vi "文字转语音.vi"(8 "错误输入（无错误）":errorcluster, 11 "textToSpeak":string="急停") -> (0 "错误输出":errorcluster)   [LabVIEW 2020]
uses:
  System.Speech
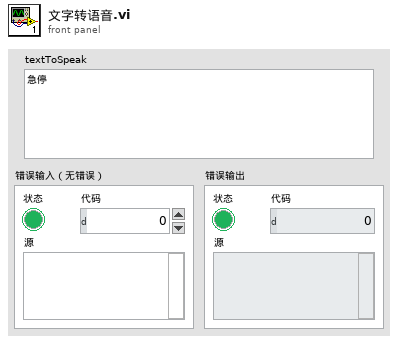
[diagram p1: front panel]
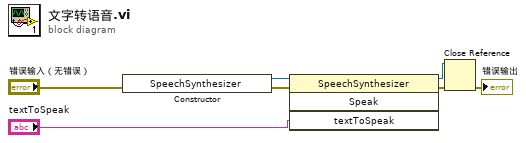
[diagram p0: block diagram]
diagram:
  n1 = constructor class="SpeechSynthesizer"(error in="错误输入（无错误）") -> (reference out=w7:refnum<k24>, error out=w3:errorcluster)  [unwired: 2 in, 1 out]
  n2 = invoke class="SpeechSynthesizer" method="Speak"(reference=w7, error in=w3, "textToSpeak"="textToSpeak") -> (reference out=w4:refnum<k24>, error out=w5:errorcluster)  [unwired: 1 in, 2 out]
  n3 = Close Reference(reference=w4, error in (no error)=w5) -> (error out=→"错误输出":errorcluster)
